vi "tcpserver.vi"() -> ()   [LabVIEW 2021]
panel:
  in  "Stop":bool
  out "Waveform Graph":dbl[](graph)
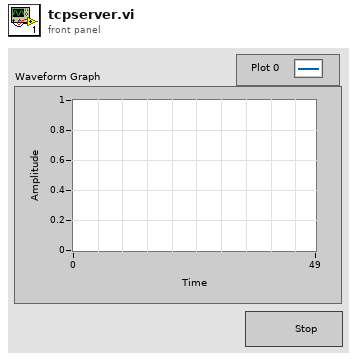
[diagram p1: front panel]
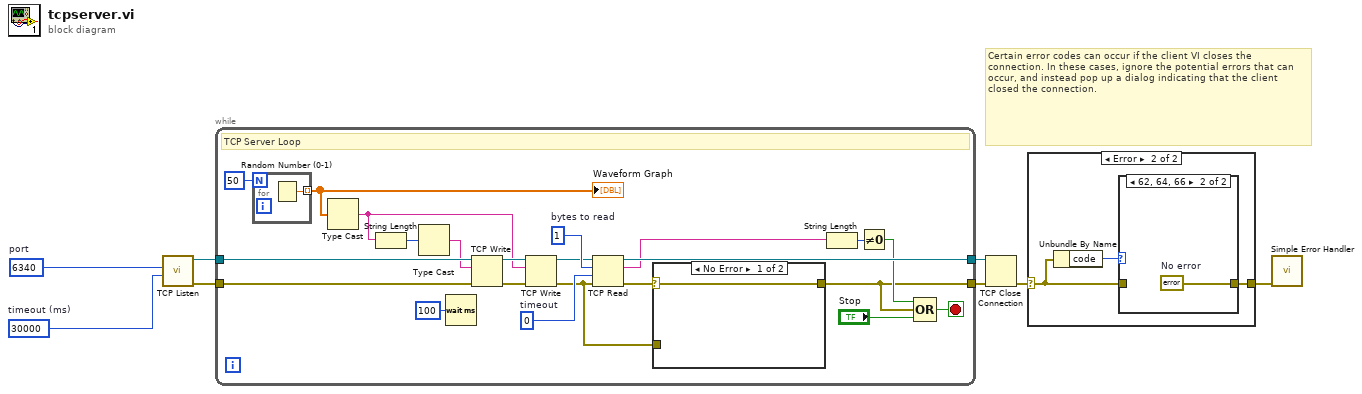
[diagram p0: block diagram]
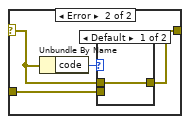
[diagram p4: hidden frame]
diagram:
  w1 = u16 6340  # port
  w2 = 30000  # timeout (ms)
  # "Certain error codes can occur if the client VI closes the connection. In these cases, ignore the potential errors that can occur, and instead pop up a dialog indicating that the client closed the connection."
  n1 = call <vilib>:"TCP Listen.vi"("timeout ms (wait forever: -1)"=w2, "port"=w1) -> ("error out"=w3:errorcluster, "connection ID"=w4:refnum<k5>)  [unwired: 5 in, 3 out]
  n2 = while {
    tunnel: [w10] -> w7
    tunnel: [w16] -> w8
    tunnel: w4 -> [w30]
    tunnel: w3 -> [w21]
    stop <- w23 stop-if-true
    w15 = 0  # timeout
    w18 = 1  # bytes to read
    # "TCP Server Loop"
    n3 = for {
      N: 50 ("# of Points") -> [_]
      tunnel: [w38] -> w19 mode=indexing
      n4 = Random Number (0-1)() -> (number: 0 to 1=w38:dbl)
    }
    "Waveform Graph" <- w19
    n5 = Type Cast(x=w19) -> (*(type *) &x=w25:string)  [unwired: 1 out]
    n6 = String Length(string=w25) -> (length=w27:i32)
    n7 = Type Cast(x=w27) -> (*(type *) &x=w26:string)  [unwired: 1 out]
    n8 = Wait (ms)(milliseconds to wait=u32 100) -> ()  [unwired: 1 out]
    n9 = TCP Write(connection ID=w30, data in=w26, error in (no error)=w21) -> (connection ID out=w29:refnum<k5>, error out=w28:errorcluster)  [unwired: 2 out]
    n10 = TCP Write(connection ID=w29, data in=w25, error in (no error)=w28) -> (connection ID out=w17:refnum<k5>, error out=w9:errorcluster)  [unwired: 2 out]
    n11 = TCP Read(connection ID=w17, bytes to read=w18, error in (no error)=w9, 9:w15) -> (connection ID out=w16:refnum<k5>, data out=w13:string, error out=w11:errorcluster)  [unwired: 1 out]
    n12 = case shown="No Error" w11 {
      selector: w11 -> [w31 w34]
      tunnel: [w31 w32] -> w10
      tunnel: w9 -> [_ w33]
      frame No Error {
      }
      frame Error {
        n13 = Unbundle By Name(w34) -> ("code"=w35:i32)
        n14 = case shown="Default" w35 {
          tunnel: w34 -> [w36 _]
          tunnel: w33 -> [_ w37]
          tunnel: [w36 w37] -> w32
          frame Default {
          }
          frame 56 {
          }
        }
      }
    }
    n15 = String Length(string=w13) -> (length=w14:i32)
    n16 = Not Equal To 0?(x=w14) -> (x != 0?=w12:bool)
    n17 = Compound Arithmetic op=OR(w12, w10, "Stop") -> (w23:bool)
  }
  n18 = TCP Close Connection(connection ID=w8, error in (no error)=w7) -> (error out=w6:errorcluster)  [unwired: 2 out]
  n19 = case shown="Error" w6 {
    selector: w6 -> [w39 w41]
    tunnel: [w39 w40] -> w5
    frame No Error {
    }
    frame Error {
      n20 = Unbundle By Name(w41) -> ("code"=w42:i32)
      n21 = case shown="62, 64, 66" w42 {
        tunnel: w41 -> [w43 _]
        tunnel: [w43 w44] -> w40
        frame Default {
        }
        frame 62, 64, 66 {
          w44 = errorcluster {"status"=FALSE, "code"=0, "source"=""}  # No error
        }
      }
    }
  }
  n22 = call <vilib>:"Simple Error Handler.vi"("error in (no error)"=w5) -> ()  [unwired: 1 in, 8 out]
